vi "Example_OE1311&1351 Control.vi"() -> ()   [LabVIEW 2011]
uses:
  <vilib>/Utility/error.llb/DialogType.ctl
panel:
  out "loss count":i32=-1
  in  "Sample count":u32
  in  "buffer":u8
  out "Zero Data?":bool
  out "Queue out":errorcluster caption="error out"
  out "Queue output":refnum<queue>
  in  "Timeout":u32=100
  in  "Port":u32=10001
  in  "IP Address":string
  out "Freq":dbl
  out "xita":dbl
  out "R":dbl
  out "Input Overlaod":bool
  out "PLL Lock":bool
  out "Error":string
  out "Serial Versions":string
  in  "Table":T1(tab) caption="选项卡控件"
  in  "OE1300_Configure Input Filter":T2 {"Input Coupling" items=["AC", "DC"]; "Input Source" items=["A", "B", "Current"]}
  in  "OE1300_Configure Ref Phase":T3={"Reference Source"=0, "Internal Frequency(Hz)"=1000.0, "Phase  (degree)"=0.0, "External Ref Trigger"=0, "Instrument Mode "=4} {"Instrument Mode" items=["OE1311"=3, "OE1351"=4, "OE1301"=5]; "External Ref Trigger" items=["TTL Rising Edge", "TTL Fallling Edge", "Sine Zero Crossing"]; "Phase  (degree)" min=-180.0 max=180.0 format="%#.2g"; "Internal Frequency(Hz)" min=0.001 max=1002000.0 format="%#.3f"; "Reference Source" items=["External", "Internal", "Self"]}
  in  "OE1300_Configure Sens and Filter":T4={"Time Constant(s) "=0.1, "Low Pass Filter Slope "=1, "Enable Sync Filter "=0, "Input Range"=2} {"Input Range" items=["5 V/uA", "2 V/uA", "1 V/uA", "500 mV/nA", "200 mV/nA", "100 mV/nA", "50 mV/nA", "20 mV/nA", "10 mV/nA", "5 mV/nA", "2 mV/nA", "1 mV/nA", "500 uV/pA", "200 uV/pA", "100 uV/pA", "50 uV/pA", "20 uV/pA", "10 uV/pA", "5 uV/pA", "2 uV/pA", "1 uV/pA", "500 nV/fA", "200 nV/fA", "100 nV/fA", "50 nV/fA", "20 nV/fA", "10 nV/fA", "5 nV/fA", "2 nV/fA", "1 nV/fA"]; "Enable Sync Filter" items=["OFF", "ON"]; "Low Pass Filter Slope" items=["6 dB/oct", "12 dB/oct", "18 db/oct", "24 dB/oct", "30 dB/oct", "36 dB/oct", "42 dB/oct", "48 dB/oct"]; "Time Constant(s)" min=1e-06 max=3000.0}
  in  "OE1300_Configure Channel Out":T5={"CH2 Offset"=0.0, "CH1 Offset"=0.0, "CH2 Expand"=1, "CH1 Expand"=1, "AUX OUT1"=1.0, "AUX OUT2"=1.0, "CH 1"=3, "CH 2"=3} {"CH 2" items=["Fixed", "X", "Y", "R", "Theta", "Xh1", "Yh1", "Rh1", "Theta h1", "Xh2", "Yh2", "Rh2", "Theta h2", "Xh3", "Yh3", "Rh3", "Theta h3", "Rh4", "Xh4", "Yh4", "Theta h4", "Rh5", "Xh5", "Yh5", "Theta h5", "Rh6", "Xh6", "Yh6", "Theta h6", "Rh7", "Xh6", "Yh6", "Theta h7", "X_Noise", "Y_Noise", "Freq", "AuxIn1", "AuxIn2"]; "CH 1" items=["Fixed", "X", "Y", "R", "Theta", "Xh1", "Yh1", "Rh1", "Theta h1", "Xh2", "Yh2", "Rh2", "Theta h2", "Xh3", "Yh3", "Rh3", "Theta h3", "Rh4", "Xh4", "Yh4", "Theta h4", "Rh5", "Xh5", "Yh5", "Theta h5", "Rh6", "Xh6", "Yh6", "Theta h6", "Rh7", "Xh6", "Yh6", "Theta h7", "X_Noise", "Y_Noise", "Freq", "AuxIn1", "AuxIn2"]; "AUX OUT2" min=-10.0 max=10.0 format="%#.3g"; "AUX OUT1" min=-10.0 max=10.0 format="%#.3g"; "CH1 Expand" min=1 max=256; "CH2 Expand" min=1 max=256; "CH1 Offset" min=-100.0 max=100.0 format="%#.2g"; "CH2 Offset" min=-100.0 max=100.0 format="%#.2g"}
  in  "OE1300_Configure Sine Out":T6={"Sine Output Amplitude (V)"=0.1, "SineOut Mode"=0} {"SineOut Mode" items=["OFF", "Fixed"]; "Sine Output Amplitude (V)" min=0.0001 max=5.0 format="%#.4g"}
  in  "OE1300_Configure Demodulator":T7={"Demodulator"=1, "Mode"=0, "Arbitrary Frequency"=1000.0, "Harmonic"=1, "Instrument Mode "=4, "Phase  (degree)"=0.0} {"Phase  (degree)" min=-180.0 max=180.0 format="%#.2g"; "Instrument Mode" items=["OE1311"=3, "OE1351"=4, "OE1301"=5]; "Harmonic" min=1 max=32767; "Arbitrary Frequency" min=1e-06 max=1002000.0 format="%#.3f"; "Mode" items=["Harm", "Arb_Freq"]; "Demodulator" items=["1", "2", "3", "4", "5", "6", "7"]}
  in  "Save Button":bool
  in  "file path":path
  in  "Sample Rate":dbl=0.1 min=0.001 max=100.0
  out "Status":string
  in  "Connect":bool
  in  "VISA resource name":refnum<visa-resource-name>
  in  "Remote Mode":u16(ring)=1 items=["RS232"=1, "Ethernet"=3]
  in  "Baud Rate (115200)":u32=115200
  # "Tel          :   +86-020-84133345\nWebsite  :   www.ssi-instrument.com\nE-mail     :   support@si-instrument.com"
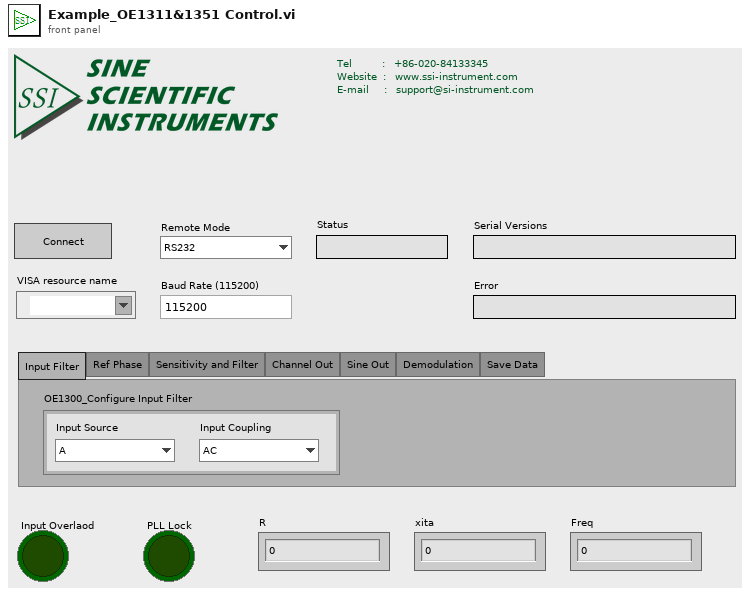
[diagram p1: front panel]
types:
  T1 = enum32{"Input Filter", "Ref Phase", "Sensitivity and Filter", "Channel Out", "Sine Out", "Demodulation", "Save Data"}
  T2 = cluster{"Input Source":u16, "Input Coupling ":u16}
  T3 = cluster{"Reference Source":u16, "Internal Frequency(Hz)":dbl, "Phase  (degree)":dbl, "External Ref Trigger":u16, "Instrument Mode ":u16}
  T4 = cluster{"Time Constant(s) ":dbl, "Low Pass Filter Slope ":u8, "Enable Sync Filter ":u16, "Input Range":u16}
  T5 = cluster{"CH2 Offset":dbl, "CH1 Offset":dbl, "CH2 Expand":i16, "CH1 Expand":i16, "AUX OUT1":dbl, "AUX OUT2":dbl, "CH 1":u16, "CH 2":u16}
  T6 = cluster{"Sine Output Amplitude (V)":dbl, "SineOut Mode":u8}
  T7 = cluster{"Demodulator":u16, "Mode":u16, "Arbitrary Frequency":dbl, "Harmonic":u16, "Instrument Mode ":u16, "Phase  (degree)":dbl}
  T8 = enum16{"OE1022", "OE1022D", "OE1201", "OE2031&OE2041", "OE1311&OE1351"}
  T9 = cluster{"Port":u32, "Timeout":u32, "IP Address":string}
  T10 = cluster{"PLL Lock(1: External Lock)":bool, "Input Overlaod":bool}
  T11 = cluster{"X":dbl, "Y":dbl, "R":dbl, "θ":dbl, "XD1":dbl, "YD1":dbl, "RD1":dbl, "θD1":dbl, "XD2":dbl, "YD2":dbl, "RD2":dbl, "θD2":dbl, "XD3":dbl, "YD3":dbl, "RD3":dbl, "θD3":dbl, "XD4":dbl, "YD4":dbl, "RD4":dbl, "θD4":dbl, "XD5":dbl, "YD5":dbl, "RD5":dbl, "θD5":dbl, "XD6":dbl, "YD6":dbl, "RD6":dbl, "θD6":dbl, "XD7":dbl, "YD7":dbl, "RD7":dbl, "θD7":dbl, "X-Noise":dbl, "Y-Noise":dbl, "Frequency":dbl, "AUX-IN1":dbl, "AUX-IN2":dbl}
  T12 = typedef "DialogType.ctl" = u16
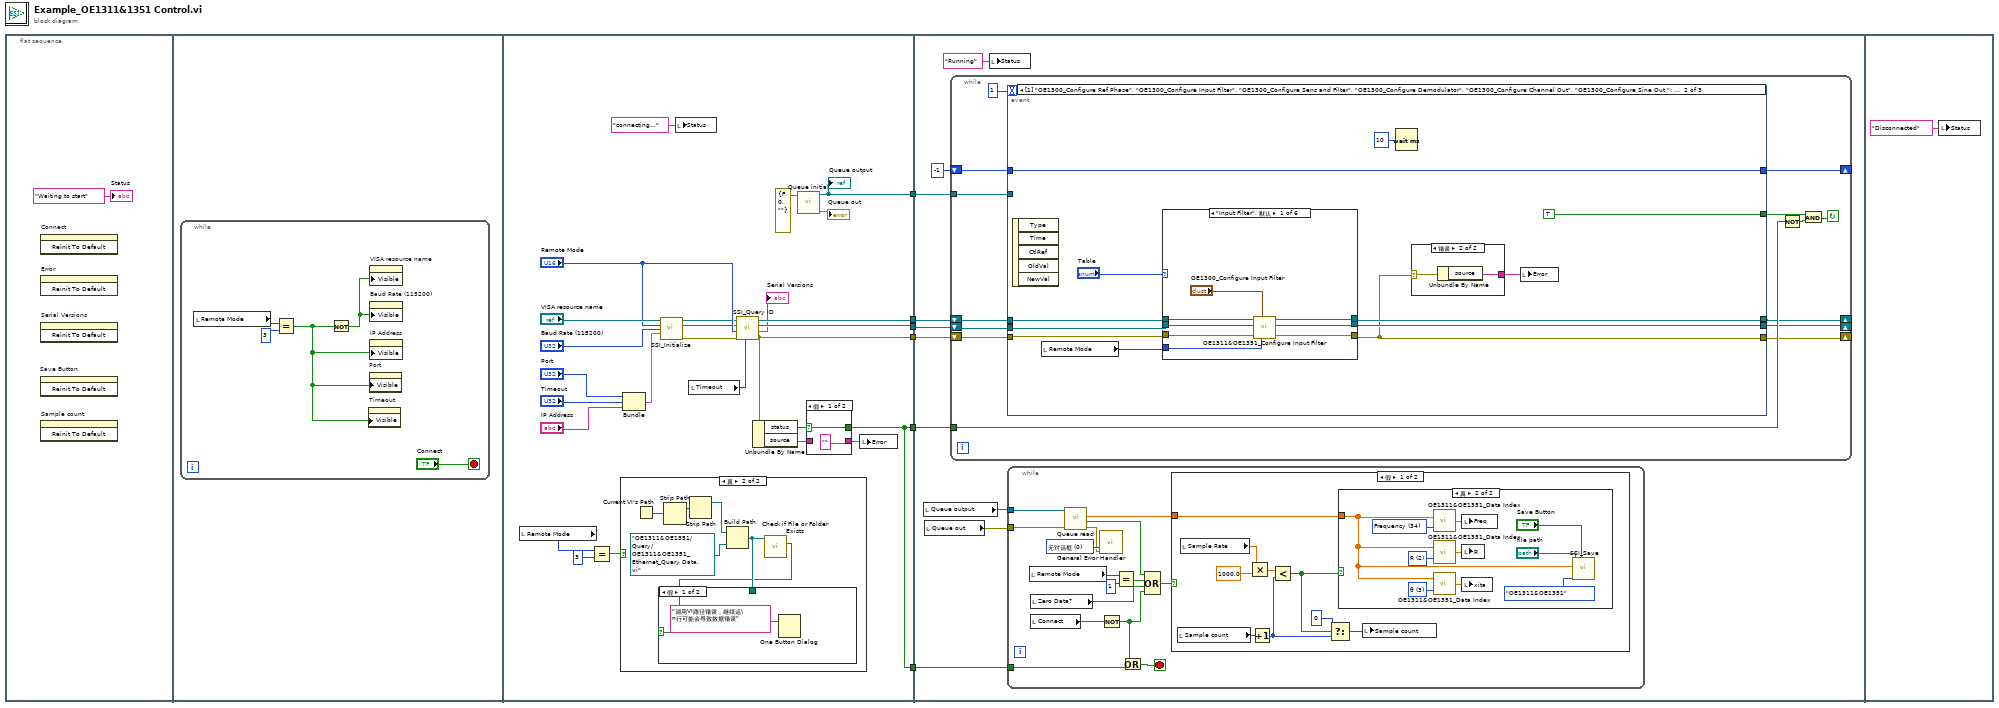
[diagram p0: block diagram]
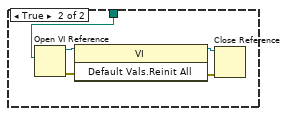
[diagram p3: hidden frame]
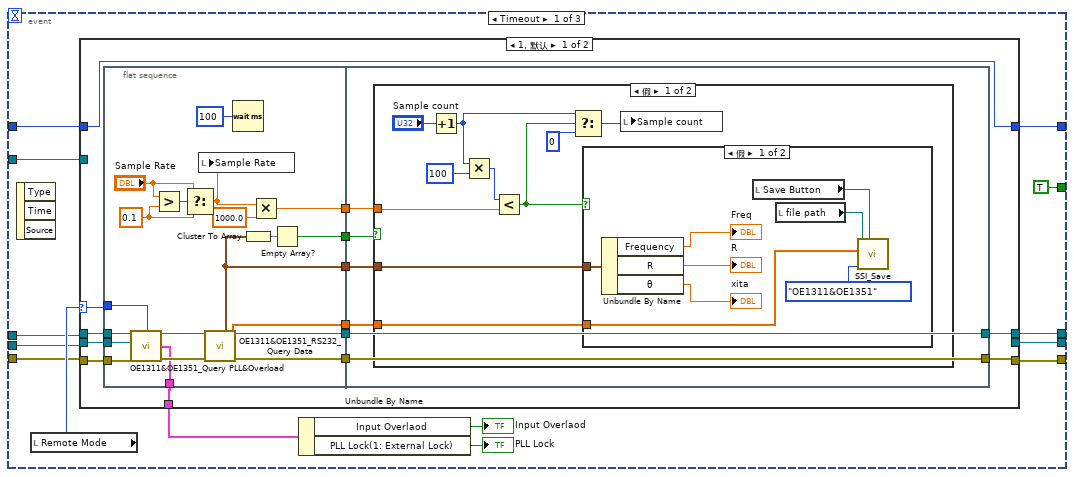
[diagram p7: hidden frame]
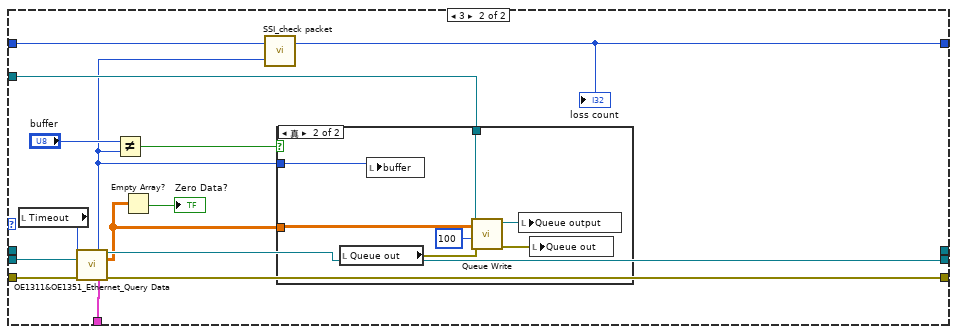
[diagram p10: hidden frame]
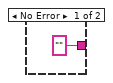
[diagram p12: hidden frame]
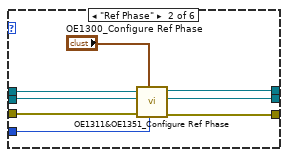
[diagram p13: hidden frame]
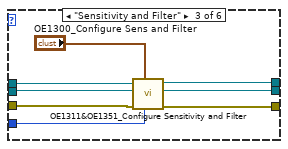
[diagram p14: hidden frame]
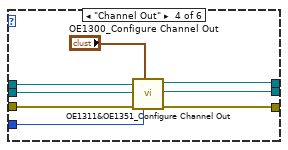
[diagram p15: hidden frame]
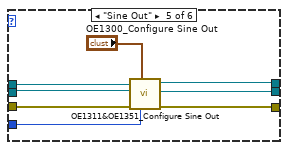
[diagram p16: hidden frame]
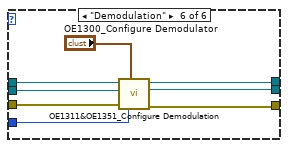
[diagram p17: hidden frame]
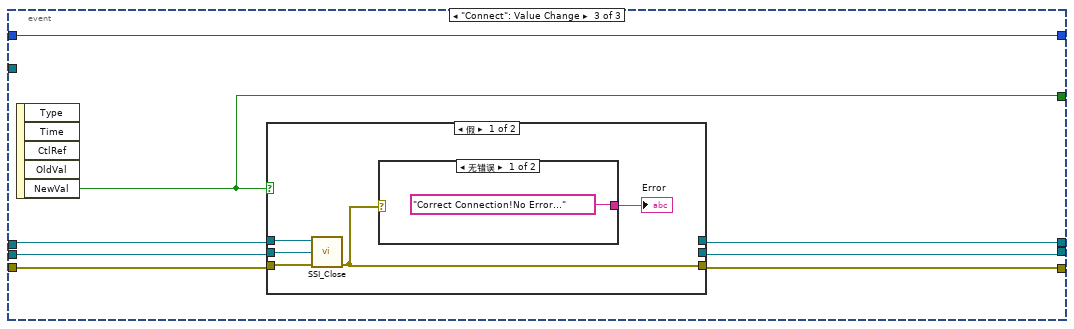
[diagram p18: hidden frame]
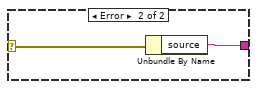
[diagram p19: hidden frame]
diagram:
  n1 = flat-sequence {
    tunnel: [w35] -> w6
    tunnel: [w34] -> w5
    tunnel: [w31] -> w4
    tunnel: [w19] -> w3
    tunnel: [w21] -> w2
    tunnel: [w19] -> w1
    tunnel: w6 -> [w63]
    tunnel: w5 -> [w62]
    tunnel: w4 -> [w61]
    tunnel: w3 -> [w60]
    tunnel: w2 -> [w57]
    tunnel: w1 -> [w55]
    frame #0 {
      n2 = invoke on="Save Button" class="Bool (严格)" method="Reinit To Default"() -> ()  [unwired: 3 in, 3 out]
      n3 = invoke on="Connect" class="Bool (严格)" method="Reinit To Default"() -> ()  [unwired: 3 in, 3 out]
      n4 = invoke on="Error" class="Str" method="Reinit To Default"() -> ()  [unwired: 3 in, 3 out]
      n5 = invoke on="Serial Versions" class="Str" method="Reinit To Default"() -> ()  [unwired: 3 in, 3 out]
      n6 = invoke on="Sample count" class="DigNum (严格)" method="Reinit To Default"() -> ()  [unwired: 3 in, 3 out]
      "Status" <- "Waiting to start" ("status")
    }
    frame #1 {
      n7 = while {
        stop <- "Connect" stop-if-true
        n8 = local read "Remote Mode"() -> (w10:u16)
        n9 = Equal?(x=w10, y=u16 3) -> (x = y?=w11:bool)
        n10 = Not(x=w11) -> (.not. x?=w8:bool)
        n11 = property on="Timeout" class="DigNum (严格)"("Visible"=w11) -> ()  [unwired: 2 in, 2 out]
        n12 = property on="Port" class="DigNum (严格)"("Visible"=w11) -> ()  [unwired: 2 in, 2 out]
        n13 = property on="VISA resource name" class="VISAName"("Visible"=w8) -> ()  [unwired: 2 in, 2 out]
        n14 = property on="Baud Rate (115200)" class="DigNum (严格)"("Visible"=w8) -> ()  [unwired: 2 in, 2 out]
        n15 = property on="IP Address" class="Str"("Visible"=w11) -> ()  [unwired: 2 in, 2 out]
      }
    }
    frame #2 {
      n16 = local read "Remote Mode"() -> (w15:u16)
      n17 = Equal?(x=w15, y=u16 3) -> (x = y?=w13:bool)
      n18 = case shown="真" w13 {
        frame False {
        }
        frame True {
          n19 = Current VI's Path() -> (path=w40:path)
          n20 = Strip Path(path=w40) -> (stripped path=w39:path)  [unwired: 1 out]
          n21 = Strip Path(path=w39) -> (stripped path=w41:path)  [unwired: 1 out]
          n22 = Build Path(base path=w41, name or relative path=path "OE1311&OE1351/Query/OE1311&OE1351_Ethernet_Query Data.vi") -> (appended path=w44:path)
          n23 = call <vilib>:"Check if File or Folder Exists.vi"("path"=w44) -> ("file or folder exists?"=w42:bool)  [unwired: 8 in, 2 out]
          n24 = case shown="假" w42 {
            tunnel: w44 -> [_ w50]
            frame False {
              n25 = One Button Dialog(message="调用VI路径错误，继续运\n行可能会导致数据错误" ("消息")) -> ()  [unwired: 1 in, 1 out]
            }
            frame True {
              n26 = Open VI Reference(vi path=w50) -> (vi reference=w47:refnum<vi>, error out=w46:errorcluster)  [unwired: 5 in]
              n27 = invoke class="VI" method="Default Vals.Reinit All"(reference=w47, error in=w46) -> (reference out=w49:refnum<vi>, error out=w48:errorcluster)  [unwired: 1 in, 1 out]
              n28 = Close Reference(reference=w49, error in (no error)=w48) -> ()  [unwired: 1 out]
            }
          }
        }
      }
      n29 = Bundle("Port"="Port", "Timeout"="Timeout", "IP Address"="IP Address") -> (w26:T9)  [unwired: 1 in]
      n30 = call "SSI_Initialize.vi"("VISA resource name"="VISA resource name", "Remote Mode"="Remote Mode", "baud rate (921600)"="Baud Rate (115200)", "Ethernet"=w26) -> ("VISA resource name out"=w16:refnum<visa-resource-name>, "connection ID(Ethernet)"=w17:refnum<k5>, "error out"=w18:errorcluster)  [unwired: 9 in]
      n31 = local write "Status"("connecting..." ("status")) -> ()
      n32 = local read "Timeout"() -> (w24:u32)
      n33 = call "SSI_Query ID.vi"("Timeout"=w24, "Error in (no error)"=w18, "Remote Mode"="Remote Mode", "Connection ID in"=w17, "VISA resource name"=w16) -> ("Error out"=w31:errorcluster, "Read Buffer"=→"Serial Versions":string, "Connection ID out"=w34:refnum<k5>, "VISA resource  out"=w35:refnum<visa-resource-name>)  [unwired: 3 in]
      n34 = Unbundle By Name(w31) -> ("status"=w32:bool, "source"=w30:string)
      n35 = call "Queue initial.vi"("Error in (no error)"=errorcluster {"status"=FALSE, "code"=0, "source"=""}) -> ("Error out"=→"Queue out":errorcluster, "Queue output"=w21:refnum<queue>)  [unwired: 9 in]
      "Queue output" <- w21
      n36 = case shown="假" w32 {
        selector: w32 -> [w52 w54]
        tunnel: [w52 w54] -> w19
        tunnel: ["" w53] -> w29
        tunnel: w30 -> [_ w53]
        frame False {
        }
        frame True {
        }
      }
      n37 = local write "Error"(w29) -> ()
    }
    frame #3 {
      n38 = local read "Queue output"() -> (w59:refnum<queue>)
      n39 = local read "Queue out"() -> (w58:errorcluster)
      n40 = while {
        tunnel: w60 -> [w108]
        tunnel: w57 -> [w104]
        shift-right: [w101] -> _
        shift-left: w63 -> [w107]
        shift-right: [w102] -> _
        shift-left: w62 -> [w106]
        shift-right: [w103] -> _
        shift-left: w61 -> [w105]
        shift-right: [w99] -> _
        shift-left: -1 ("loss count") -> [w100]
        stop <- w109 continue-if-true
        n41 = event shown="[1] \"OE1300_Configure Ref Phase\", \"OE1300_Configure Input Filter\", \"OE1300_Configure Sens and Filter\", \"OE1300_Configure Demodulator\", \"OE1300_Configure Channel Out\", \"OE1300_Configure Sine Out \": 值改变" {
          selector: _ -> [_ _ _]
          dyn-events: _ -> [_ _ _]
          timeout: 1 -> [_ _ _]
          tunnel: [TRUE ("NewVal") TRUE ("Stop") w275] -> w110
          tunnel: [w126 w212 w276] -> w103
          tunnel: [w118 w216 w270] -> w101
          tunnel: [w125 w215 w271] -> w102
          tunnel: w107 -> [w122 w210 w272]
          tunnel: w106 -> [w120 w209 w273]
          tunnel: w105 -> [w121 w208 w274]
          tunnel: w104 -> [w123 _ _]
          tunnel: w100 -> [w117 w207 w269]
          tunnel: [w116 w207 w269] -> w99
          event Timeout {
            n42 = event-data() -> ()  [unwired: 1 in, 3 out]
            n43 = local read "Remote Mode"() -> (w124:u16)
            n44 = case shown="1, 默认" w124 {
              selector: w124 -> [w134 _]
              tunnel: [w136 w194] -> w126
              tunnel: [_ w197] -> w125
              tunnel: w121 -> [w140 w196]
              tunnel: w120 -> [w139 w195]
              tunnel: w122 -> [w138 _]
              tunnel: w123 -> [_ w191]
              tunnel: [w135 w188] -> w119
              tunnel: [w137 _] -> w118
              tunnel: w117 -> [w127 w187]
              tunnel: [w127 w185] -> w116
              frame 1, Default {
                n45 = flat-sequence {
                  tunnel: w134 -> [w149]
                  tunnel: [w148] -> w133
                  tunnel: [w147] -> w132
                  tunnel: [w146] -> w131
                  tunnel: [w145] -> w130
                  tunnel: [w144] -> w129
                  tunnel: [w143] -> w128
                  tunnel: [w142] -> w135
                  tunnel: w140 -> [w152]
                  tunnel: w139 -> [w151]
                  tunnel: w138 -> [w150]
                  tunnel: w133 -> [w165]
                  tunnel: w132 -> [w166]
                  tunnel: [w166] -> w137
                  tunnel: [w165] -> w136
                  tunnel: w131 -> [w164]
                  tunnel: w130 -> [w163]
                  tunnel: w129 -> [w162]
                  tunnel: w128 -> [w161]
                  frame #0 {
                    w158 = 0.1 ("y")
                    n46 = call "OE1311&OE1351_Query PLL&Overload.vi"("VISA resource name"=w150, "Connection ID in"=w151, "Remote Mode"=w149, "Error in (no error)"=w152) -> ("VISA resource  out"=w153:refnum<visa-resource-name>, "OE1300_Query PLL&Overload"=w142:T10, "Error out"=w154:errorcluster)  [unwired: 7 in, 2 out]
                    n47 = Greater?(x="Sample Rate", y=w158) -> (0:w156:bool)
                    n48 = Select(t="Sample Rate", s=w156, f=w158) -> (s? t:f=w155:dbl)
                    n49 = local write "Sample Rate"(w155) -> ()
                    n50 = call "OE1311&OE1351_RS232_Query Data.vi"("VISA resource name"=w153, "Error in (no error)"=w154) -> ("VISA resource  out"=w147:refnum<visa-resource-name>, "Data Array"=w143:dbl[], "Parameter Values"=w144:T11, "Error out"=w148:errorcluster)  [unwired: 9 in, 1 out]
                    n51 = Wait (ms)(milliseconds to wait=u32 100 ("等待时间（毫秒）")) -> ()  [unwired: 1 out]
                    n52 = Cluster To Array(cluster=w144) -> (array=w160:dbl[])
                    n53 = Multiply(x=w155, y=1000.0) -> (x*y=w145:dbl)
                    n54 = Empty Array?(array=w160) -> (empty?=w146:bool)
                  }
                  frame #1 {
                    n55 = case shown="假" w164 {
                      tunnel: w163 -> [w173 _]
                      tunnel: w162 -> [w172 _]
                      tunnel: w161 -> [w171 _]
                      frame False {
                        n56 = Increment(x="Sample count") -> (x+1=w168:u32)
                        n57 = Multiply(x=w168, y=u32 100) -> (x*y=w175:u32)
                        n58 = Less?(x=w175, y=w173) -> (x < y?=w169:bool)
                        n59 = Select(t=w168, s=w169, f=u32 0 ("Loop count variable")) -> (s? t:f=w170:u32)
                        n60 = case shown="假" w169 {
                          tunnel: w172 -> [w178 _]
                          tunnel: w171 -> [w177 _]
                          frame False {
                            n61 = Unbundle By Name(w178) -> ("Frequency"=→"Freq":dbl, "R"=→"R":dbl, "θ"=→"xita":dbl)
                            n62 = local read "Save Button"() -> (w181:bool)
                            n63 = local read "file path"() -> (w180:path)
                            n64 = call "SSI_Save.vi"("file path (dialog if empty)"=w180, "1D data"=w177, "Instrument Mode"=T8."OE1311&OE1351", "Save Button"=w181) -> ()  [unwired: 7 in]
                          }
                          frame True {
                          }
                        }
                        n65 = local write "Sample count"(w170) -> ()
                      }
                      frame True {
                      }
                    }
                  }
                }
              }
              frame 3 {
                n66 = local read "Timeout"() -> (w198:u32)
                n67 = call "OE1311&OE1351_Ethernet_Query Data.vi"("Connection ID in"=w195, "Timeout"=w198, "Error in (no error)"=w196) -> ("Buffer Count"=w186:u8, "Connection ID out"=w197:refnum<k5>, "Total Date Array"=w190:dbl[][], "PLL&Overload"=w188:T10, "Error out"=w194:errorcluster)  [unwired: 5 in, 3 out]
                n68 = Not Equal?(x="buffer", y=w186) -> (x != y?=w192:bool)
                n69 = Empty Array?(array=w190) -> (empty?=→"Zero Data?":bool)
                n70 = call "SSI_check packet.vi"("input"=w186, "input loss"=w187) -> ("loss count"=w185:i32)  [unwired: 1 out]
                "loss count" <- w185
                n71 = case shown="真" w192 {
                  tunnel: w191 -> [_ w204]
                  tunnel: w186 -> [_ w200]
                  tunnel: w190 -> [_ w199]
                  frame False {
                  }
                  frame True {
                    n72 = local read "Queue out"() -> (w201:errorcluster)
                    n73 = local write "buffer"(w200) -> ()
                    n74 = call "Queue Write.vi"("Error in (no error)"=w201, "Group Count"=100, "Input Array"=w199, "Queue Input"=w204) -> ("Error out"=w202:errorcluster, "Queue output"=w203:refnum<queue>)  [unwired: 6 in]
                    n75 = local write "Queue output"(w203) -> ()
                    n76 = local write "Queue out"(w202) -> ()
                  }
                }
              }
            }
            n77 = Unbundle By Name(w119) -> ("Input Overlaod"=→"Input Overlaod":bool, "PLL Lock(1: External Lock)"=→"PLL Lock":bool)
          }
          event "OE1300_Configure Ref Phase", "OE1300_Configure Input Filter", "OE1300_Configure Sens and Filter", "OE1300_Configure Demodulator", "OE1300_Configure Channel Out", "OE1300_Configure Sine Out": Value Change {
            n78 = event-data() -> ()  [unwired: 1 in, 5 out]
            n79 = local read "Remote Mode"() -> (w214:u16)
            n80 = case shown="\"Input Filter\", 默认" "Table" {
              tunnel: [w226 w235 w243 w249 w258 w267] -> w216
              tunnel: [w227 w234 w244 w251 w260 w266] -> w212
              tunnel: [w228 w233 w242 w250 w259 w265] -> w215
              tunnel: w214 -> [w225 w232 w240 w252 w256 w268]
              tunnel: w210 -> [w223 w231 w239 w247 w255 w263]
              tunnel: w209 -> [w221 w230 w238 w246 w254 w262]
              tunnel: w208 -> [w222 w229 w237 w245 w253 w261]
              frame "Input Filter", Default {
                n81 = call "OE1311&OE1351_Configure Input Filter.vi"("OE1300_Configure Input Filter"="OE1300_Configure Input Filter", "Error in (no error)"=w222, "Remote Mode"=w225, "Connection ID in"=w221, "VISA resource name"=w223) -> ("Error out"=w227:errorcluster, "Connection ID out"=w228:refnum<k5>, "VISA resource  out"=w226:refnum<visa-resource-name>)  [unwired: 3 in, 1 out]
              }
              frame "Ref Phase" {
                n82 = call "OE1311&OE1351_Configure Ref Phase.vi"("OE1300_Configure Ref Phase"="OE1300_Configure Ref Phase", "Error in (no error)"=w229, "Remote Mode"=w232, "Connection ID in"=w230, "VISA resource name"=w231) -> ("Error out"=w234:errorcluster, "Connection ID out"=w233:refnum<k5>, "VISA resource  out"=w235:refnum<visa-resource-name>)  [unwired: 3 in, 1 out]
              }
              frame "Sensitivity and Filter" {
                n83 = call "OE1311&OE1351_Configure Sensitivity and Filter.vi"("OE1300_Configure \nSens and Filter"="OE1300_Configure Sens and Filter", "Error in (no error)"=w237, "Remote Mode"=w240, "Connection ID in"=w238, "VISA resource name"=w239) -> ("Error out"=w244:errorcluster, "Connection ID out"=w242:refnum<k5>, "VISA resource  out"=w243:refnum<visa-resource-name>)  [unwired: 3 in, 1 out]
              }
              frame "Channel Out" {
                n84 = call "OE1311&OE1351_Configure Channel Out.vi"("OE1300_Configure Channel Out"="OE1300_Configure Channel Out", "Error in (no error)"=w245, "Remote Mode"=w252, "Connection ID in"=w246, "VISA resource name"=w247) -> ("Error out"=w251:errorcluster, "Connection ID out"=w250:refnum<k5>, "VISA resource  out"=w249:refnum<visa-resource-name>)  [unwired: 3 in, 1 out]
              }
              frame "Sine Out" {
                n85 = call "OE1311&OE1351_Configure Sine Out.vi"("OE1300_Configure Sine Out"="OE1300_Configure Sine Out", "Error in (no error)"=w253, "Remote Mode"=w256, "Connection ID in"=w254, "VISA resource name"=w255) -> ("Error out"=w260:errorcluster, "Connection ID out"=w259:refnum<k5>, "VISA resource  out"=w258:refnum<visa-resource-name>)  [unwired: 3 in, 1 out]
              }
              frame "Demodulation" {
                n86 = call "OE1311&OE1351_Configure Demodulation.vi"("OE1300_Configure Demodulator"="OE1300_Configure Demodulator", "Error in (no error)"=w261, "Remote Mode"=w268, "Connection ID in"=w262, "VISA resource name"=w263) -> ("Error out"=w266:errorcluster, "Connection ID out"=w265:refnum<k5>, "VISA resource  out"=w267:refnum<visa-resource-name>)  [unwired: 3 in, 1 out]
              }
            }
            n87 = Wait (ms)(milliseconds to wait=u32 10 ("等待时间（毫秒）")) -> ()  [unwired: 1 out]
            n88 = case shown="错误" w212 {
              selector: w212 -> [_ w220]
              tunnel: ["" ("source") w219] -> w211
              frame No Error {
              }
              frame Error {
                n89 = Unbundle By Name(w220) -> ("source"=w219:string)
              }
            }
            n90 = local write "Error"(w211) -> ()
          }
          event "Connect": Value Change {
            n91 = event-data() -> ("NewVal"=w275:bool)  [unwired: 1 in, 4 out]
            n92 = case shown="假" w275 {
              tunnel: [w281 w287] -> w276
              tunnel: w274 -> [w279 w287]
              tunnel: w273 -> [w278 w286]
              tunnel: w272 -> [w277 w285]
              tunnel: [_ w286] -> w271
              tunnel: [_ w285] -> w270
              frame False {
                n93 = call "SSI_Close.vi"("Error in (no error)"=w279, "Connection ID in"=w278, "VISA resource name"=w277) -> ("Error out"=w281:errorcluster)  [unwired: 4 in]
                n94 = case shown="无错误" w281 {
                  selector: w281 -> [_ w284]
                  tunnel: ["Correct Connection!No Error..." ("source") w283] -> w280
                  frame No Error {
                  }
                  frame Error {
                    n95 = Unbundle By Name(w284) -> ("source"=w283:string)
                  }
                }
                "Error" <- w280
              }
              frame True {
              }
            }
          }
        }
        n96 = Not(x=w108) -> (.not. x?=w111:bool)
        n97 = And(x=w110, y=w111) -> (x .and. y?=w109:bool)
      }
      n98 = local write "Status"("Running" ("status")) -> ()
      n99 = while {
        tunnel: w59 -> [w72]
        tunnel: w58 -> [w71]
        tunnel: w55 -> [w67]
        stop <- w65 stop-if-true
        w74 = T12 0 items=["无对话框", "确定信息", "继续或停止信息", "确定信息＋警告", "继续/停止+警告"] ("type of dialog (OK msg:1)")
        n100 = local read "Remote Mode"() -> (w79:u16)
        n101 = local read "Zero Data?"() -> (w75:bool)
        n102 = local read "Connect"() -> (w70:bool)
        n103 = call "Queue read.vi"("Error in (no error)"=w71, "Queue Input"=w72) -> ("Error out"=w73:errorcluster, "Timeout？"=w68:bool, "Output Array"=w69:sgl[])  [unwired: 7 in]
        n104 = call <vilib>:"General Error Handler.vi"("type of dialog (OK msg:1)"=w74, "error in (no error)"=w73) -> ()  [unwired: 9 in, 5 out]
        n105 = Not(x=w70) -> (.not. x?=w66:bool)
        n106 = Equal?(x=w79, y=u16 1) -> (x = y?=w76:bool)
        n107 = Or(x=w66, y=w67) -> (x .or. y?=w65:bool)
        n108 = Compound Arithmetic op=OR(w68, w76, w75, w66) -> (w77:bool)
        n109 = case shown="假" w77 {
          tunnel: w69 -> [w88 _]
          frame False {
            n110 = local read "Sample count"() -> (w85:u32)
            n111 = local read "Sample Rate"() -> (w87:dbl)
            n112 = Multiply(x=w87, y=1000.0) -> (x*y=w84:dbl)
            n113 = Increment(x=w85) -> (x+1=w80:u32)
            n114 = Less?(x=w84, y=w80) -> (x < y?=w83:bool)
            n115 = Select(t=u32 0 ("Loop count variable"), s=w83, f=w80) -> (s? t:f=w82:u32)
            n116 = case shown="真" w83 {
              tunnel: w88 -> [_ w94]
              frame False {
              }
              frame True {
                w89 = u16 3 items=["X", "Y", "R", "θ", "XD1", "YD1", "RD1", "θD1", "XD2", "YD2", "RD2", "θD2", "XD3", "YD3", "RD3", "θD3", "XD4", "YD4", "RD4", "θD4", "XD5", "YD5", "RD5", "θD5", "XD6", "YD6", "RD6", "θD6", "XD7", "YD7", "RD7", "θD7", "X_Noise", "Y_Noise", "Frequency", "AUX-IN1", "AUX-IN2"] ("Parameter Type")
                w90 = u16 2 items=["X", "Y", "R", "θ", "XD1", "YD1", "RD1", "θD1", "XD2", "YD2", "RD2", "θD2", "XD3", "YD3", "RD3", "θD3", "XD4", "YD4", "RD4", "θD4", "XD5", "YD5", "RD5", "θD5", "XD6", "YD6", "RD6", "θD6", "XD7", "YD7", "RD7", "θD7", "X_Noise", "Y_Noise", "Frequency", "AUX-IN1", "AUX-IN2"] ("Parameter Type")
                w91 = u16 34 items=["X", "Y", "R", "θ", "XD1", "YD1", "RD1", "θD1", "XD2", "YD2", "RD2", "θD2", "XD3", "YD3", "RD3", "θD3", "XD4", "YD4", "RD4", "θD4", "XD5", "YD5", "RD5", "θD5", "XD6", "YD6", "RD6", "θD6", "XD7", "YD7", "RD7", "θD7", "X_Noise", "Y_Noise", "Frequency", "AUX-IN1", "AUX-IN2"] ("Parameter Type")
                n117 = call "OE1311&OE1351_Data Index.vi"("Parameter Type"=w91, "Input Date Array"=w94) -> ("Parameter"=w95:dbl)
                n118 = call "OE1311&OE1351_Data Index.vi"("Parameter Type"=w90, "Input Date Array"=w94) -> ("Parameter"=w93:dbl)
                n119 = call "OE1311&OE1351_Data Index.vi"("Parameter Type"=w89, "Input Date Array"=w94) -> ("Parameter"=w92:dbl)
                n120 = local write "Freq"(w95) -> ()
                n121 = local write "R"(w93) -> ()
                n122 = local write "xita"(w92) -> ()
                n123 = call "SSI_Save.vi"("file path (dialog if empty)"="file path", "1D data"=w94, "Instrument Mode"=T8."OE1311&OE1351", "Save Button"="Save Button") -> ()  [unwired: 7 in]
              }
            }
            n124 = local write "Sample count"(w82) -> ()
          }
          frame True {
          }
        }
      }
    }
    frame #4 {
      n125 = local write "Status"("Disconnected" ("status")) -> ()
    }
  }
